vi "Binary Search on One Hot Encoded Number (U64)_pipeleined.vi"(9 "Input Valid":bool=TRUE, 10 "One Hot encoded Number":u64 format="%064b") -> (1 "Output Valid":bool=TRUE, 2 "Binary Number":u8, 5 "Leading One Position":bool[](array[boolean]))   [LabVIEW 2011]
doc: "<b> Latency = 5 Ticks </b>"
uses:
  <vilib>/rvi/FXPMathLib/basic elements/FxpDiscreteDelay/XNode/nifxpmath_DiscreteDelay.xnode
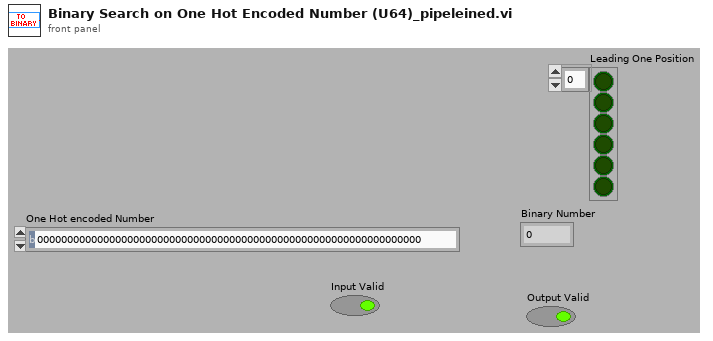
[diagram p1: front panel]
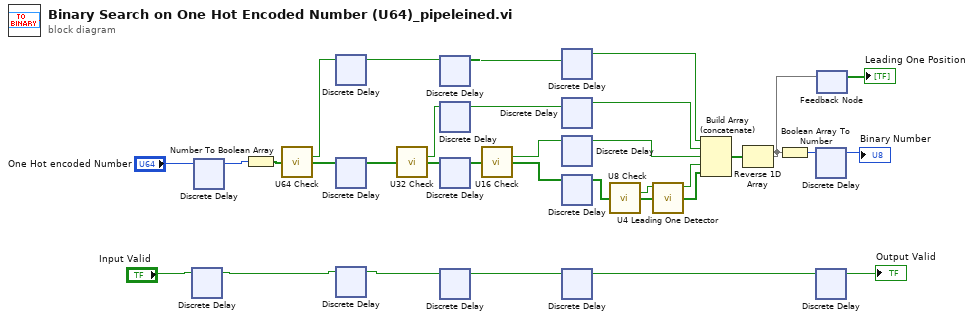
[diagram p0: block diagram]
diagram:
  n1 = xnode "Discrete Delay"("D"="Input Valid") -> ("Q"=w8:bool)
  n2 = xnode "Discrete Delay"("D"="One Hot encoded Number") -> ("Q"=w10:u64)
  n3 = Number To Boolean Array(number=w10) -> (Boolean array=w1:bool[])
  n4 = call <userlib>:"U64 Check.vi"("64--bit array"=w1) -> ("Lower Half has one?"=w24:bool, "Half with one?"=w32:bool[])  [unwired: 13 in]
  n5 = xnode "Discrete Delay"("D"=w24) -> ("Q"=w20:bool)
  n6 = xnode "Discrete Delay"("D"=w32) -> ("Q"=w19:bool[])
  n7 = xnode "Discrete Delay"("D"=w8) -> ("Q"=w22:bool)
  n8 = call <userlib>:"U32 Check.vi"("32-bit array"=w19) -> ("Lower Half has one?"=w25:bool, "Half with one?"=w31:bool[])  [unwired: 13 in]
  n9 = xnode "Discrete Delay"("D"=w20) -> ("Q"=w16:bool)
  n10 = xnode "Discrete Delay"("D"=w25) -> ("Q"=w17:bool)
  n11 = xnode "Discrete Delay"("D"=w31) -> ("Q"=w18:bool[])
  n12 = xnode "Discrete Delay"("D"=w22) -> ("Q"=w21:bool)
  n13 = call <userlib>:"U16 Check.vi"("16-bit array"=w18) -> ("Lower Half has one?"=w26:bool, "Half with one?"=w30:bool[])  [unwired: 13 in]
  n14 = xnode "Discrete Delay"("D"=w16) -> ("Q"=w12:bool)
  n15 = xnode "Discrete Delay"("D"=w17) -> ("Q"=w13:bool)
  n16 = xnode "Discrete Delay"("D"=w26) -> ("Q"=w14:bool)
  n17 = xnode "Discrete Delay"("D"=w30) -> ("Q"=w15:bool[])
  n18 = xnode "Discrete Delay"("D"=w21) -> ("Q"=w5:bool)
  n19 = call <userlib>:"U8 Check.vi"("8-bit array"=w15) -> ("Lower Half has one?"=w27:bool, "Half with one?"=w29:bool[])  [unwired: 13 in]
  n20 = call <userlib>:"U4 Leading One Detector.vi"("4-Bit Array"=w29) -> ("Leading One Position"=w28:bool[])  [unwired: 14 in]
  n21 = Build Array (concatenate)(w12, w13, w14, w27, w28) -> (w23:bool[])
  n22 = Reverse 1D Array(array=w23) -> (reversed array=w3:bool[])
  n23 = Boolean Array To Number(Boolean array=w3) -> (number=w7:u8)
  n24 = xnode "Discrete Delay"("D"=w7) -> ("Q"=→"Binary Number":u8)
  n25 = xnode "Discrete Delay"("D"=w5) -> ("Q"=→"Output Valid":bool)
  n26 = feedback-in #1(w3) -> ()
  n27 = feedback #1() -> (→"Leading One Position":bool[])  [unwired: 1 in]
